vi "子VI-计算分辨率后的值.vi"(7 "测量结果":dbl[][](array[numeric]), 9 "图像X向分辨率（mm/像素）":dbl, 10 "图像Y向分辨率（mm/像素）":dbl) -> (1 "初始化的数组":dbl[][](array[numeric]))   [LabVIEW 2018]
panel:
  out "测量结果 2":dbl[](array[numeric])
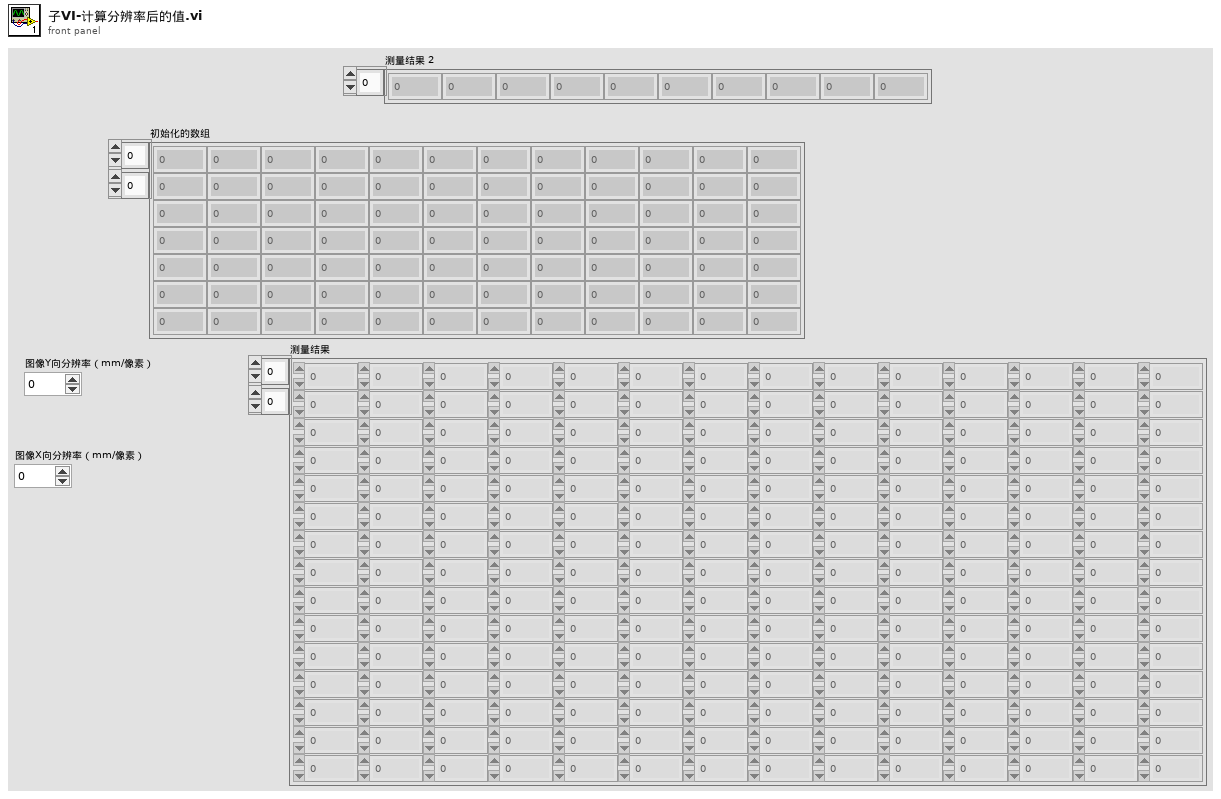
[diagram p1: front panel]
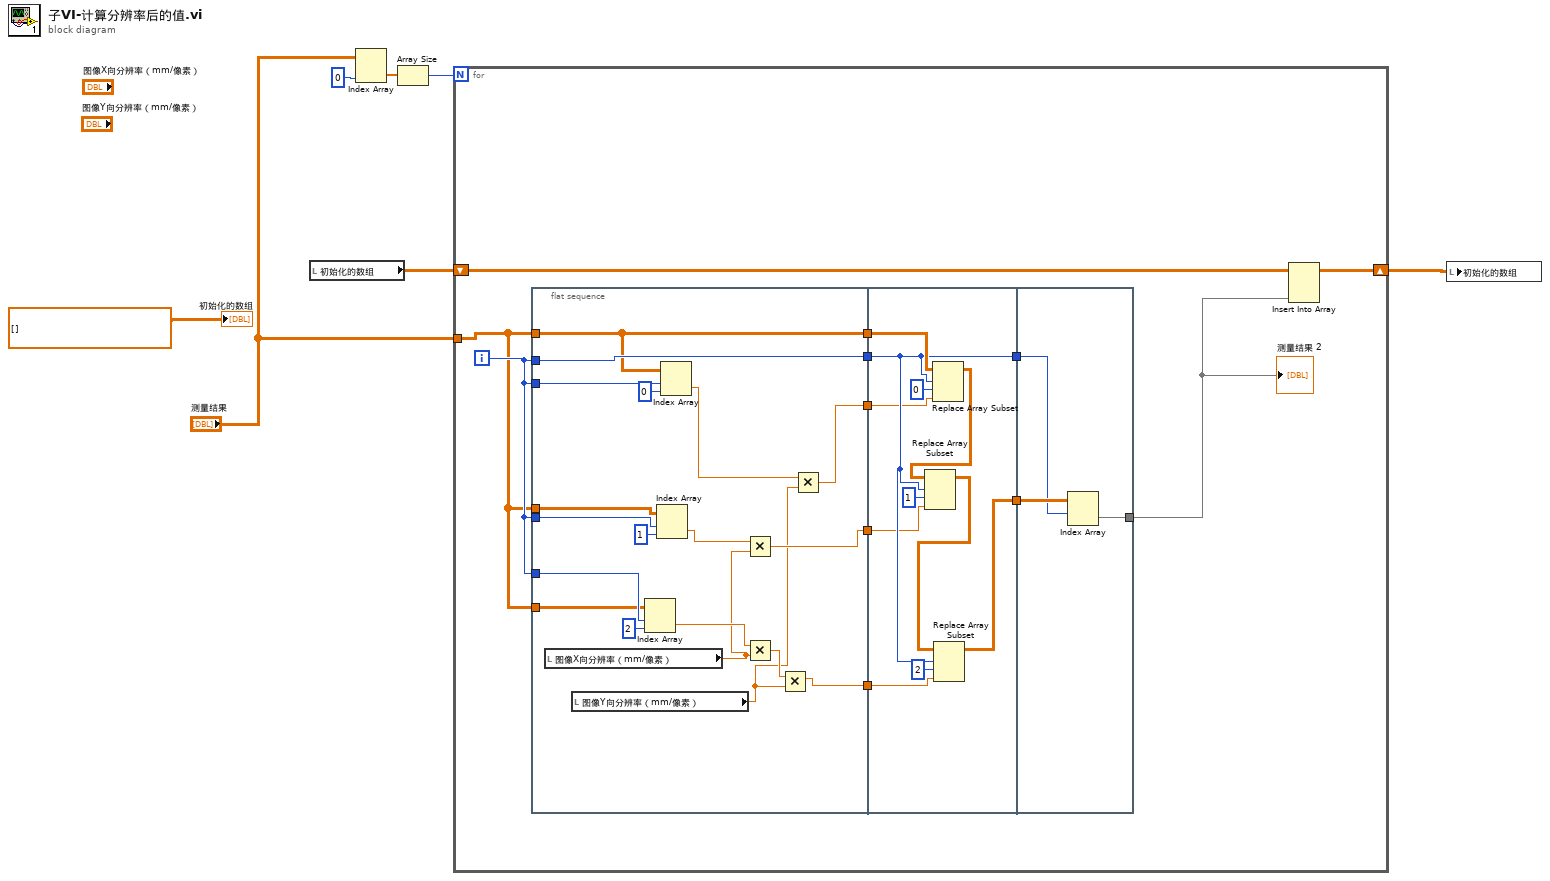
[diagram p0: block diagram]
diagram:
  n1 = local read "初始化的数组"() -> (w2:dbl[][])
  n2 = Index Array(array="测量结果", index (col)=0 ("禁用的索引 (列)")) -> (element=w5:dbl[])  [unwired: 1 in]
  n3 = Array Size(array=w5) -> (size(s)=w6:i32)
  n4 = for {
    N: w6 -> [_]
    tunnel: "测量结果" -> [w11]
    shift-right: [w15] -> w1
    shift-left: w2 -> [w16]
    i -> [w12]
    n5 = flat-sequence {
      tunnel: w11 -> [w34]
      tunnel: w12 -> [w38]
      tunnel: [w34] -> w19
      tunnel: w12 -> [w36]
      tunnel: [w36] -> w18
      tunnel: w12 -> [w33]
      tunnel: w12 -> [w31]
      tunnel: w11 -> [w30]
      tunnel: w11 -> [w29]
      tunnel: [w26] -> w10
      tunnel: [w22] -> w9
      tunnel: [w24] -> w8
      tunnel: w19 -> [w47]
      tunnel: w18 -> [w43]
      tunnel: [w43] -> w17
      tunnel: [w41] -> w14
      tunnel: w10 -> [w44]
      tunnel: w9 -> [w40]
      tunnel: w8 -> [w39]
      tunnel: w17 -> [w51]
      tunnel: w14 -> [w52]
      tunnel: [w50] -> w13
      frame #0 {
        n6 = local read "图像X向分辨率（mm/像素）"() -> (w20:dbl)
        n7 = local read "图像Y向分辨率（mm/像素）"() -> (w21:dbl)
        n8 = Index Array(array=w30, index (row)=w31, index (col)=2 ("禁用的索引 (列)")) -> (element=w28:dbl)
        n9 = Index Array(array=w29, index (row)=w33, index (col)=1 ("禁用的索引 (列)")) -> (element=w25:dbl)
        n10 = Index Array(array=w34, index (row)=w38, index (col)=0 ("禁用的索引 (列)")) -> (element=w23:dbl)
        n11 = Multiply(x=w25, y=w20) -> (x*y=w24:dbl)
        n12 = Multiply(x=w28, y=w20) -> (x*y=w27:dbl)
        n13 = Multiply(x=w27, y=w21) -> (x*y=w26:dbl)
        n14 = Multiply(x=w23, y=w21) -> (x*y=w22:dbl)
      }
      frame #1 {
        n15 = Replace Array Subset(array=w47, new element=w40, index (row)=w43, index (col)=0 ("禁用的索引 (列)")) -> (w46:dbl[][])
        n16 = Replace Array Subset(array=w46, new element=w39, index (row)=w43, index (col)=1 ("禁用的索引 (列)")) -> (w42:dbl[][])
        n17 = Replace Array Subset(array=w42, new element=w44, index (row)=w43, index (col)=2 ("禁用的索引 (列)")) -> (w41:dbl[][])
      }
      frame #2 {
        n18 = Index Array(array=w52, index (row)=w51) -> (element=w50:dbl[])  [unwired: 1 in]
      }
    }
    n19 = Insert Into Array(array=w16, new element=w13) -> (w15:dbl[][])  [unwired: 2 in]
    "测量结果 2" <- w13
  }
  n20 = local write "初始化的数组"(w1) -> ()
  "初始化的数组" <- dbl[][] [] ("初始化的数组")
